vi "Tosca-Visual Display.vi"() -> ()   [LabVIEW 2020]
uses:
  Tosca-Visual Display Queue Data.ctl
  Tosca-Visual Display Action.ctl
  Tosca-Grating.ctl
  Tosca-Grating Type.ctl
  epl-vi-lib/Utility VIs/Array Manipulation VIs/Array-Dimensions (2D).vi
  <vilib>/picture/picture.llb/Draw True-Color Pixmap.vi
panel:
  out "picture":picture
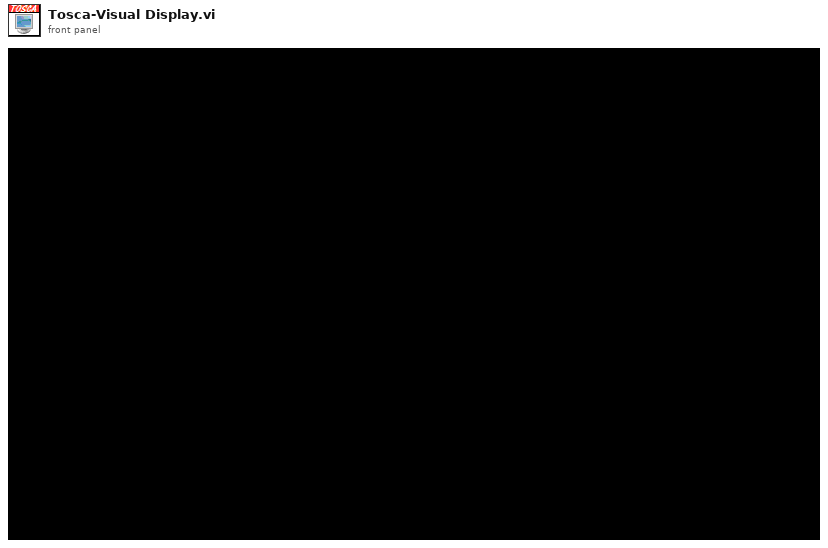
[diagram p1: front panel]
types:
  T1 = typedef "Tosca-Visual Display Queue Data.ctl" = cluster{"Action":T2, "Grating":T3}
  T2 = typedef "Tosca-Visual Display Action.ctl" = enum16{"NOOP", "Quit", "Buffer", "Draw", "Clear"}
  T3 = typedef "Tosca-Grating.ctl" = cluster{"Type":T4, "Orientation (deg)":dbl, "Spatial frequency (cpd)":dbl, "Velocity (Hz)":dbl, "Contrast":dbl, "Background intensity":dbl, "Duration (ms)":dbl, "Phase (cycles)":dbl}
  T4 = typedef "Tosca-Grating Type.ctl" = enum16{"OFF", "Square", "Sine"}
  T5 = typedef "Tosca-Visual Display Settings.ctl" = cluster{"Use PTB":bool, "IP Address":string, "Port":i32, "rect":cluster{"left":i16, "top":i16, "width":i16, "height":i16}, "Full screen":bool, "Open at start":bool, "Monitor":i32, "Monitor size (in)":dbl, "Monitor dist (in)":dbl, "Photodiode Square":cluster{"size":i16, "location":enum16{"Bottom Left", "Top Left", "Top Right", "Bottom Right"}}, "Background":dbl}
  T6 = typedef "LVRectTypeDef.ctl" = cluster{"Left":i16, "Top":i16, "Right":i16, "Bottom":i16}
  T7 = typedef "LVPointTypeDef.ctl" = cluster{"Horizontal":i16, "Vertical":i16}
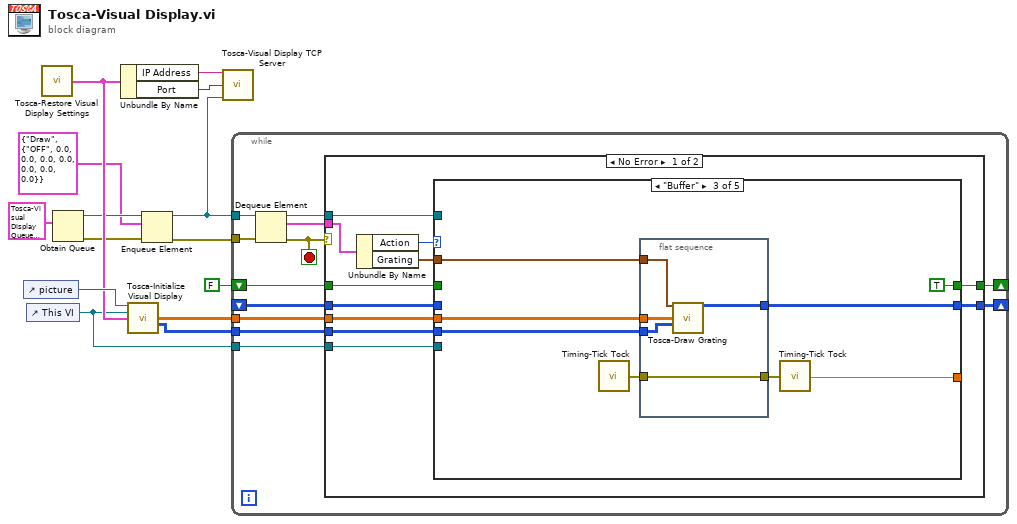
[diagram p0: block diagram]
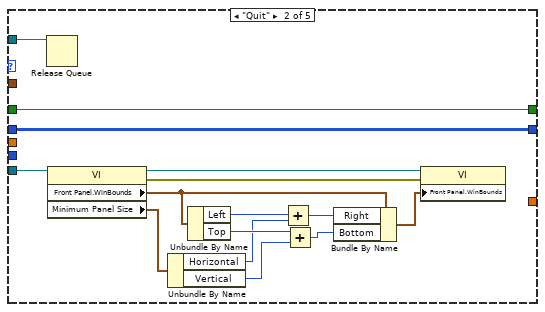
[diagram p3: hidden frame]
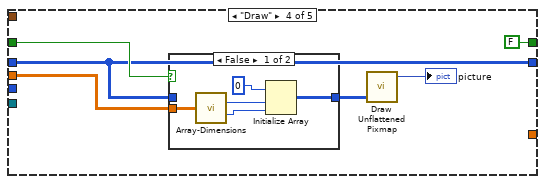
[diagram p4: hidden frame]
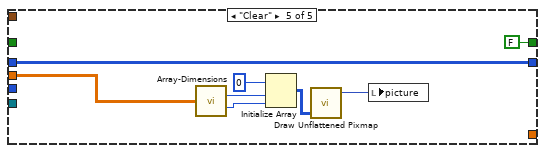
[diagram p6: hidden frame]
diagram:
  n1 = control-ref of="picture"() -> (w14:refnum<vi>)
  n2 = control-ref of="This VI"() -> (w9:refnum<vi>)
  n3 = call "Tosca-Restore Visual Display Settings.vi"() -> ("Visual Display Settings"=w13:T5)  [unwired: 14 in, 1 out]
  n4 = Obtain Queue(element data type=T1 {"Action"=enum."NOOP", "Grating"={"Type"=enum."OFF", "Orientation (deg)"=0.0, "Spatial frequency (cpd)"=0.0, "Velocity (Hz)"=0.0, "Contrast"=0.0, "Background intensity"=0.0, "Duration (ms)"=0.0, "Phase (cycles)"=0.0}}) -> (queue out=w5:refnum<queue>, error out=w4:errorcluster)  [unwired: 4 in, 1 out]
  n5 = Unbundle By Name(w13) -> ("IP Address"=w12:string, "Port"=w11:i32)
  n6 = call "Tosca-Initialize Visual Display.vi"("Picture in"=w14, "This VI"=w9, "Visual Display Settings"=w13) -> ("Array"=w8:cdb[][], "photodiode mask"=w1:u8[][])  [unwired: 10 in, 1 out]
  n7 = Enqueue Element(queue=w5, element=T1 {"Action"=enum."Draw", "Grating"={"Type"=enum."OFF", "Orientation (deg)"=0.0, "Spatial frequency (cpd)"=0.0, "Velocity (Hz)"=0.0, "Contrast"=0.0, "Background intensity"=0.0, "Duration (ms)"=0.0, "Phase (cycles)"=0.0}}, error in (no error)=w4) -> (queue out=w6:refnum<queue>, error out=w3:errorcluster)  [unwired: 1 in, 1 out]
  n8 = call "Tosca-Visual Display TCP Server.vi"("Address"=w12, "Port"=w11, "Queue"=w6) -> ()  [unwired: 12 in, 1 out]
  n9 = while {
    tunnel: w3 -> [w23]
    tunnel: w6 -> [w22]
    tunnel: w9 -> [w21]
    tunnel: w8 -> [w20]
    shift-right: [w19] -> _
    shift-left: _ -> [w18]
    shift-right: [w16] -> _
    shift-left: FALSE -> [w17]
    tunnel: w1 -> [w15]
    stop <- w26 stop-if-true
    n10 = Dequeue Element(queue=w22, error in (no error)=w23) -> (queue out=w25:refnum<queue>, element=w24:T1, error out=w26:errorcluster)  [unwired: 1 in, 1 out]
    n11 = case shown="No Error" w26 {
      tunnel: w25 -> [w35 _]
      tunnel: w24 -> [w37 _]
      tunnel: w21 -> [w34 _]
      tunnel: w20 -> [w32 _]
      tunnel: [w31 w89] -> w19
      tunnel: w18 -> [w30 w89]
      tunnel: w17 -> [w29 w88]
      tunnel: [w28 w88] -> w16
      tunnel: w15 -> [w27 _]
      frame No Error {
        n12 = Unbundle By Name(w37) -> ("Action"=w36:T2, "Grating"=w33:T3)
        n13 = case shown="\"Buffer\"" w36 {
          tunnel: w35 -> [_ w42 _ _ _]
          tunnel: w34 -> [_ w43 _ _ _]
          tunnel: w33 -> [_ _ w62 _ _]
          tunnel: w32 -> [_ _ w61 w68 w84]
          tunnel: [w39 w41 w60 w71 w86] -> w31
          tunnel: w30 -> [w39 w41 _ w71 w86]
          tunnel: w29 -> [w38 w40 _ w73 _]
          tunnel: [w38 w40 TRUE FALSE FALSE] -> w28
          tunnel: [_ _ w56 _ _] -> _
          tunnel: w27 -> [_ _ w55 _ _]
          frame "NOOP", Default {
          }
          frame "Quit" {
            n14 = Release Queue(queue=w42) -> ()  [unwired: 2 in, 3 out]
            n15 = property class="VI"(reference=w43) -> (reference out=w44:refnum<vi>, error out=w45:errorcluster, "Front Panel.WinBounds"=w49:T6, "Minimum Panel Size"=w46:T7)  [unwired: 1 in]
            n16 = Unbundle By Name(w46) -> ("Horizontal"=w48:i16, "Vertical"=w53:i16)
            n17 = Unbundle By Name(w49) -> ("Left"=w47:i16, "Top"=w52:i16)
            n18 = Add(x=w47, y=w48) -> (x+y=w50:i16)
            n19 = Add(x=w52, y=w53) -> (x+y=w54:i16)
            n20 = Bundle By Name(cluster=w49, "Right"=w50, "Bottom"=w54) -> (w51:T6)
            n21 = property class="VI"(reference=w44, error in=w45, "Front Panel.WinBounds"=w51) -> ()  [unwired: 2 out]
          }
          frame "Buffer" {
            n22 = call "Timing-Tick Tock.vi"() -> ("error out"=w58:errorcluster)  [unwired: 6 in, 1 out]
            n23 = flat-sequence {
              tunnel: w62 -> [w67]
              tunnel: w61 -> [w66]
              tunnel: [w65] -> w60
              tunnel: w58 -> [w64]
              tunnel: [w64] -> w57
              tunnel: w55 -> [w63]
              frame #0 {
                n24 = call "Tosca-Draw Grating.vi"("Grating"=w67, "Array"=w66, "photodiode mask"=w63) -> ("RGB"=w65:u32[][])  [unwired: 12 in]
              }
            }
            n25 = call "Timing-Tick Tock.vi"("error in (no error)"=w57) -> ("Elapsed time (ms)"=w56:dbl)  [unwired: 5 in, 1 out]
          }
          frame "Draw" {
            n26 = case shown="False" w73 {
              tunnel: w71 -> [_ w79]
              tunnel: [w74 w79] -> w70
              tunnel: w68 -> [w78 _]
              frame False {
                n27 = call-poly "Array-Dimensions.vi"("2D Array"=w78) -> ("# rows"=w77:i32, "# columns"=w76:i32)  [unwired: 13 in]
                n28 = Initialize Array(u32 0, w77, w76) -> (w74:u32[][])
              }
              frame True {
              }
            }
            n29 = call-poly <vilib>:"Draw Unflattened Pixmap.vi"("data (RGB format)"=w70) -> ("new picture"=→"picture":picture)  [unwired: 8 in]
          }
          frame "Clear" {
            n30 = call-poly "Array-Dimensions.vi"("2D Array"=w84) -> ("# rows"=w83:i32, "# columns"=w82:i32)  [unwired: 13 in]
            n31 = Initialize Array(u32 0, w83, w82) -> (w85:u32[][])
            n32 = call-poly <vilib>:"Draw Unflattened Pixmap.vi"("data (RGB format)"=w85) -> ("new picture"=w80:picture)  [unwired: 8 in]
            n33 = local write "picture"(w80) -> ()
          }
        }
      }
      frame Error {
      }
    }
  }
